vi "value2freq_limit_VAC.vi"(2 "Voltage [V]":dbl, 3 "Frequnecy [Hz]":dbl, 4 "Limit type (none)":T1(ring)) -> (0 "Limitation necessary":bool, 1 "Limited frequency [V]":dbl)   [LabVIEW 2020, in "Datron D4xxx.lvlib"]
doc: "This VI returns limited frequency for entered voltage value."
uses:
  Datron D4xxx.lvlib
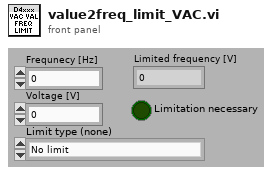
[diagram p1: front panel]
types:
  T1 = enum16{"No limit", "Always to 1kHz", "D4800", "D4805", "D4808"}
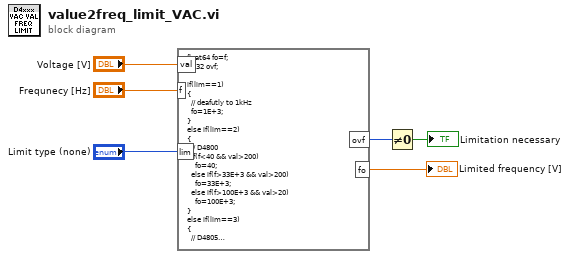
[diagram p0: block diagram]
diagram:
  n1 = formula code="float64 fo=f;\nint32 ovf;\n\nif(lim==1)\n{\n  // deafutly to 1kHz\n  fo=1E+3;\n}\nelse if(lim==2)\n{\n  // D4800\n  if(f<40 && val>200)\n    fo=40;\n  else if(f>33E+3 && val>200)\n    fo=33E+3;\n  else if(f>100E+3 && val>20)\n    fo=100E+3;\n}\nelse if(lim==3)\n{\n  // D4805\n  if(f<40 && val>200)\n    fo=40;\n  else if(f>33E+3 && val>200)\n    fo=33E+3;\n  else if(f>100E+3)\n    fo=100E+3;\n}\nelse if(lim==4)\n{\n  // D4808\n  if(f<40 && val>200)\n    fo=40;\n  else if(f>33E+3 && val>750)\n    fo=33E+3;\n  else if(f>100E+3 && val>20)\n    fo=100E+3;\n}\n\novf=f!=fo;"("val"="Voltage [V]", "f"="Frequnecy [Hz]", "lim"="Limit type (none)") -> ("ovf"=w6:i32, "fo"=→"Limited frequency [V]":dbl)
  n2 = Not Equal To 0?(x=w6) -> (x != 0?=→"Limitation necessary":bool)
